vi "Material-ConfigDialog-DiscoverPages.vi"(7 "Custom Config Pages Directory":path, 11 "error in":errorcluster) -> (4 "Configuration Dialog Page Filepaths":path[](array[path]), 6 "Display Names":string[](array[string]), 8 "Descriptions":string[](array[string]), 10 "Tree Tags":string[](array[string]), 15 "error out":errorcluster)   [LabVIEW 2013, in "Material-ConfigDialog.lvclass"]
uses:
  Material-ConfigDialog.lvclass
  Configuration Page Plugin/Pages/Plugin-001-MaterialTest.vi
  Configuration Page Plugin/Pages/Plugin-002-CalibrationTest.vi
  Deploy Application/Material-Application-Constants.vi
  Plugins/Run Material Test/Material-RunTest.lvclass
  Plugins/Run Calibration Test/Calibration-RunTest.lvclass
panel:
  # "Inputs"
  # "Outputs"
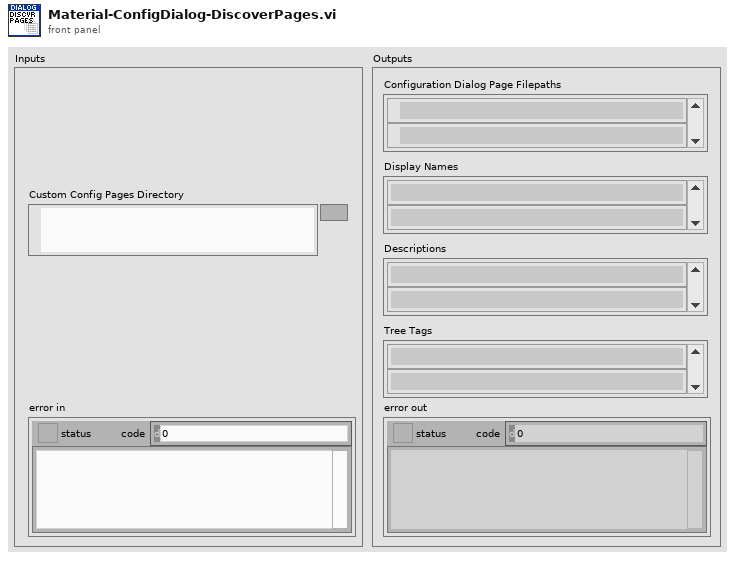
[diagram p1: front panel]
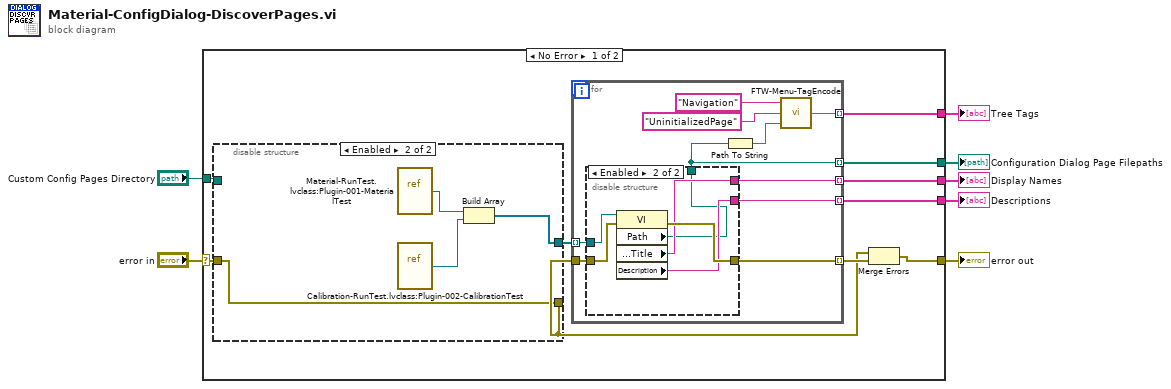
[diagram p0: block diagram]
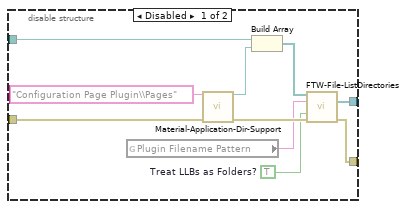
[diagram p2: hidden frame]
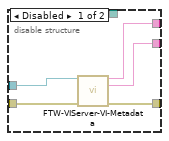
[diagram p3: hidden frame]
diagram:
  n1 = case shown="No Error" "error in" {
    selector: "error in" -> [w16 w53]
    tunnel: [w12 w53] -> w7
    tunnel: [w14 _] -> w5
    tunnel: "Custom Config Pages Directory" -> [w17 _]
    tunnel: [w11 _] -> w3
    tunnel: [w10 _] -> w2
    tunnel: [w9 _] -> w1
    frame No Error {
      n2 = disable-structure shown="Enabled" {
        disable-tunnel: w17 -> [w26 _]
        disable-tunnel: w16 -> [w25 w28]
        disable-tunnel: [w23 w28] -> w13
        disable-tunnel: [w21 w29] -> w8
        frame Disabled {
          w19 = TRUE  # Treat LLBs as Folders?
          n3 = global read "Material-Application-Constants.vi" "Plugin Filename Pattern"() -> (w18:string)
          n4 = call "Material-Application-Dir-Support.vi"("Support Resource Relative Filepath"="Configuration Page Plugin\\Pages" ("Support VI Relative Filepath"), "error in"=w25) -> ("Support Filepath"=w20:path, "error out"=w24:errorcluster)  [unwired: 12 in]
          n5 = Build Array(w26, w20) -> (w27:path[])
          n6 = call "FTW-File-ListDirectories.vi"("Directories"=w27, "Matching Filename Pattern"=w18, "Treat LLBs as Folders?"=w19, "error in"=w24) -> ("Matching Filepaths"=w21:path[], "error out"=w23:errorcluster)  [unwired: 9 in, 1 out]
        }
        frame Enabled {
          n7 = vi-ref "Material-RunTest.lvclass:Plugin-001-MaterialTest.vi"() -> (w31:refnum<vi>)
          n8 = vi-ref "Calibration-RunTest.lvclass:Plugin-002-CalibrationTest.vi"() -> (w30:refnum<vi>)
          n9 = Build Array(w31, w30) -> (w29:refnum<vi>[])
        }
      }
      n10 = for {
        tunnel: w8 -> [w33] mode=indexing
        tunnel: [w41] -> w11 mode=indexing
        tunnel: w13 -> [w40]
        tunnel: [w39] -> w15 mode=indexing
        tunnel: [w38] -> w10 mode=indexing
        tunnel: [w34] -> w9 mode=indexing
        tunnel: [w32] -> w14 mode=indexing
        n11 = disable-structure shown="Enabled" {
          disable-tunnel: [w46 w49] -> w41
          disable-tunnel: w40 -> [w45 w51]
          disable-tunnel: [w44 w50] -> w39
          disable-tunnel: [w43 w48] -> w38
          disable-tunnel: w33 -> [w42 w52]
          disable-tunnel: [_ w47] -> w32
          frame Disabled {
            n12 = call "FTW-VIServer-VI-Metadata.vi"("VI Filepath"=w42, "error in"=w45) -> ("Front Panel Title"=w46:string, "VI Description"=w43:string, "error out"=w44:errorcluster)  [unwired: 11 in]
          }
          frame Enabled {
            n13 = property class="VI"(reference=w52, error in=w51) -> (error out=w50:errorcluster, "Path"=w47:path, "Front Panel.Title"=w49:string, "Description"=w48:string)  [unwired: 1 out]
          }
        }
        n14 = Path To String(path=w32) -> (string=w36:string)
        n15 = call "FTW-Menu-TagEncode.vi"("Payload"=w36, "Command"="UninitializedPage", "Class"="Navigation") -> ("Tag"=w34:string)  [unwired: 1 in]
      }
      n16 = Merge Errors(w13, w15) -> (w12:errorcluster)
    }
    frame Error {
    }
  }
  "error out" <- w7
  "Configuration Dialog Page Filepaths" <- w5
  "Tree Tags" <- w1
  "Display Names" <- w3
  "Descriptions" <- w2
